vi "Update Measurement Details.vi"(8 "error in":errorcluster, 10 "Measurement Service Name":string, 11 "Project ref":refnum<vi>) -> (0 "error out":errorcluster)   [LabVIEW 2020, in "MeasurementService Editor.lvlib"]
uses:
  MeasurementService Editor.lvlib
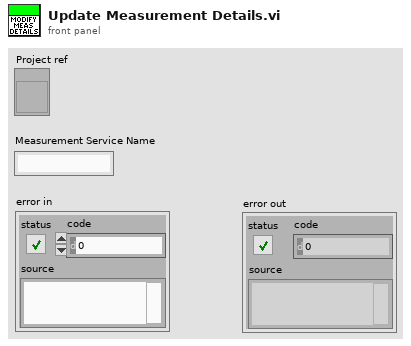
[diagram p1: front panel]
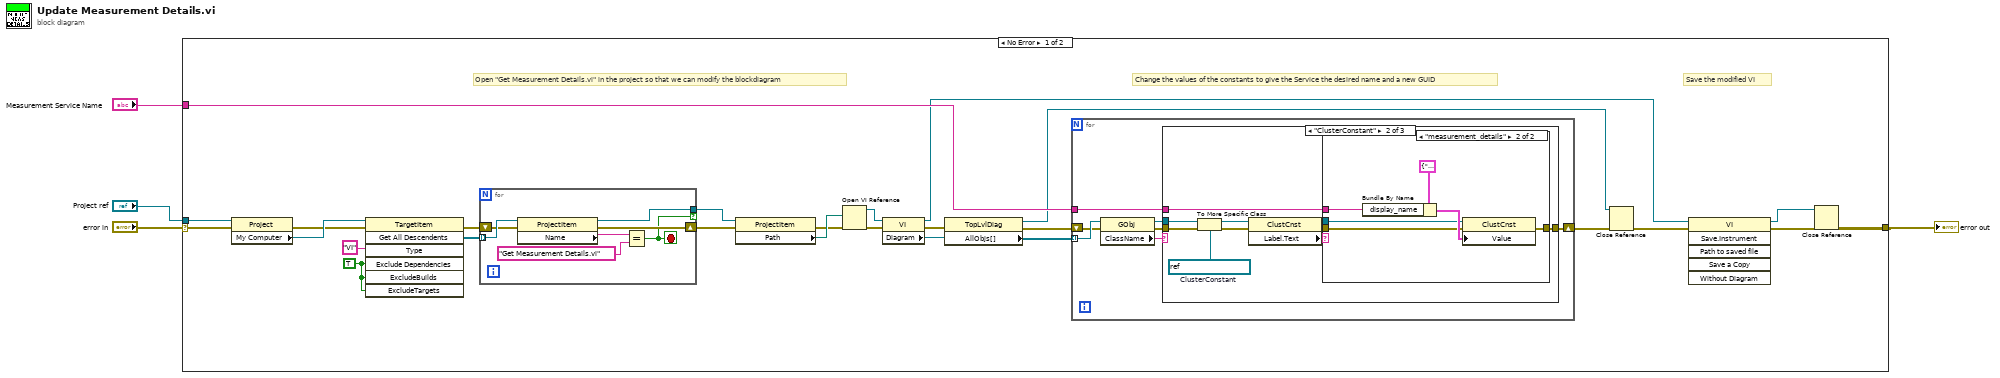
[diagram p0: block diagram]
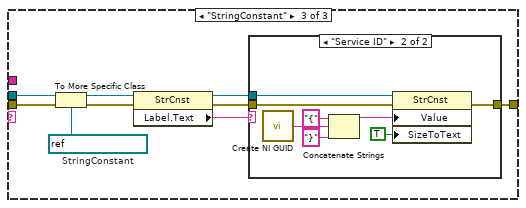
[diagram p4: hidden frame]
diagram:
  n1 = case shown="No Error" "error in" {
    selector: "error in" -> [w24 w81]
    tunnel: "Project ref" -> [w5 _]
    tunnel: [w19 w81] -> w2
    tunnel: "Measurement Service Name" -> [w10 _]
    frame No Error {
      w28 = TRUE ("ExcludeDependencies")
      # "Save the modified VI"
      # "Open \"Get Measurement Details.vi\" in the project so that we can modify the blockdiagram"
      # "Change the values of the constants to give the Service the desired name and a new GUID"
      n2 = property class="Project"(reference=w5, error in=w24) -> (error out=w25:errorcluster, "My Computer"=w26:refnum<vi>)  [unwired: 1 out]
      n3 = invoke class="TargetItem" method="Get All Descendents"(reference=w26, error in=w25, "Type"="VI", "Exclude Dependencies"=w28, "ExcludeBuilds"=w28, "ExcludeTargets"=w28) -> (error out=w30:errorcluster, "All Descendents"=w29:refnum<vi>[])  [unwired: 1 in, 5 out]
      n4 = for {
        tunnel: w29 -> [w80] mode=indexing
        shift-right: [w77] -> w21
        shift-left: w30 -> [w75]
        tunnel: [w76] -> w23 if=w74
        stop <- w74 stop-if-true
        n5 = property class="ProjectItem"(reference=w80, error in=w75) -> (reference out=w76:refnum<vi>, error out=w77:errorcluster, "Name"=w78:string)
        n6 = Equal?(x=w78, y="Get Measurement Details.vi") -> (x = y?=w74:bool)
      }
      n7 = property class="ProjectItem"(reference=w23, error in=w21) -> (error out=w20:errorcluster, "Path"=w22:path)  [unwired: 1 out]
      n8 = Open VI Reference(vi path=w22, error in (no error)=w20) -> (vi reference=w16:refnum<vi>, error out=w13:errorcluster)  [unwired: 4 in]
      n9 = property class="VI"(reference=w16, error in=w13) -> (reference out=w9:refnum<vi>, error out=w14:errorcluster, "Diagram"=w12:refnum<vi>)
      n10 = property class="TopLvlDiag"(reference=w12, error in=w14) -> (reference out=w6:refnum<vi>, error out=w11:errorcluster, "AllObjs[]"=w15:refnum<vi>[])
      n11 = for {
        tunnel: w15 -> [w37] mode=indexing
        shift-right: [w31] -> w8
        shift-left: w11 -> [w36]
        tunnel: w10 -> [w32]
        n12 = property class="GObj"(reference=w37, error in=w36) -> (reference out=w34:refnum<vi>, error out=w33:errorcluster, "ClassName"=w35:string)
        n13 = case shown="\"ClusterConstant\"" w35 {
          tunnel: w34 -> [_ w47 w63]
          tunnel: w33 -> [w38 w46 w62]
          tunnel: w32 -> [_ w45 _]
          tunnel: [w38 w44 w61] -> w31
          frame Default {
          }
          frame "ClusterConstant" {
            w48 = refnum<vi> refnum  # ClusterConstant
            n14 = To More Specific Class(target class=w48, reference=w47, error in=w46) -> (specific class reference=w43:refnum<vi>, error out=w42:errorcluster)
            n15 = property class="ClustCnst"(reference=w43, error in=w42) -> (reference out=w41:refnum<vi>, error out=w40:errorcluster, "Label.Text"=w39:string)
            n16 = case shown="\"measurement_details\"" w39 {
              tunnel: w45 -> [_ w54]
              tunnel: [w49 w53] -> w44
              tunnel: w41 -> [_ w51]
              tunnel: w40 -> [w49 w50]
              frame Default {
              }
              frame "measurement_details" {
                n17 = Bundle By Name(cluster=cluster{"display_name":string, "version":string} {"display_name"="Measurement Template", "version"="1.0.0"} ("ni_measurements_v1_MeasurementDetails"), "display_name"=w54) -> (w52:cluster{"display_name":string, "version":string})
                n18 = property class="ClustCnst"(reference=w51, error in=w50, "Value"=w52) -> (error out=w53:errorcluster)  [unwired: 1 out]
              }
            }
          }
          frame "StringConstant" {
            w64 = refnum<vi> refnum  # StringConstant
            n19 = To More Specific Class(target class=w64, reference=w63, error in=w62) -> (specific class reference=w60:refnum<vi>, error out=w59:errorcluster)
            n20 = property class="StrCnst"(reference=w60, error in=w59) -> (reference out=w57:refnum<vi>, error out=w56:errorcluster, "Label.Text"=w58:string)
            n21 = case shown="\"Service ID\"" w58 {
              tunnel: [w65 w73] -> w61
              tunnel: w57 -> [_ w68]
              tunnel: w56 -> [w65 w67]
              frame Default {
              }
              frame "Service ID" {
                n22 = call <vilib>:"Create NI GUID.vi"() -> ("NI GUID"=w72:string)
                n23 = Concatenate Strings("{" ("string"), w72, "}" ("string")) -> (w69:string)
                n24 = property class="StrCnst"(reference=w68, error in=w67, "Value"=w69, "SizeToText"=TRUE ("Size To Text?")) -> (error out=w73:errorcluster)  [unwired: 1 out]
              }
            }
          }
        }
      }
      n25 = Close Reference(reference=w6, error in (no error)=w8) -> (error out=w7:errorcluster)
      n26 = invoke class="VI" method="Save.Instrument"(reference=w9, error in=w7) -> (reference out=w18:refnum<vi>, error out=w17:errorcluster)  [unwired: 4 in, 4 out]
      n27 = Close Reference(reference=w18, error in (no error)=w17) -> (error out=w19:errorcluster)
    }
    frame Error {
    }
  }
  "error out" <- w2
